vi "SetIndividualJoints.vi"(0 "Mode":T1=1 items=["Position"=1, "Velocity"=2, "Effort"=3], 1 "node":string, 2 "Joint States":T2(array[cluster]), 3 "error in":errorcluster) -> (6 "error out":errorcluster)   [LabVIEW 2012]
doc: "Set individual joints on Baxter"
uses:
  <userlib>/ROSforLV/ROS/Code/SubVIs/JointMode.ctl
  <userlib>/ROSforLV/ROS/Code/SubVIs/BaxterSide.ctl
  <userlib>/ROSforLV/ROS/Code/Console/Servers/ServerSubs/TopicDef.ctl
  <userlib>/ROSforLV/ROS/Code/SubVIs/_ROSDirection.ctl
  <userlib>/ROSforLV/ROS/MessageBuilding/std_msgs/subs/i32Scalar.vi
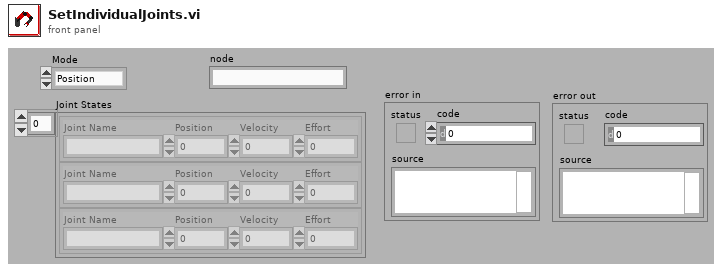
[diagram p1: front panel]
types:
  T1 = typedef "JointMode.ctl" = u8
  T2 = cluster{"Joint Name":string, "Position":dbl, "Velocity":dbl, "Effort":dbl}[]
  T3 = typedef "BaxterSide.ctl" = enum16{"left", "right"}
  T4 = typedef "TopicDef.ctl" = cluster{"Topic":string, "Type":string, "Action":T5, "Update (ms)":u16, "queue size":u16}
  T5 = typedef "_ROSDirection.ctl" = enum16{"Node", "Publisher", "Subscriber", "ServiceClient", "ServiceProvider"}
  T6 = typedef "_ROSControl.ctl" = cluster{"topic port":u16, "Node":string, "topic":string, "type":string, "node port":u16, "error ":errorcluster, "Direction":T5, "Update (ms)":u16, "FIFO size":u16}
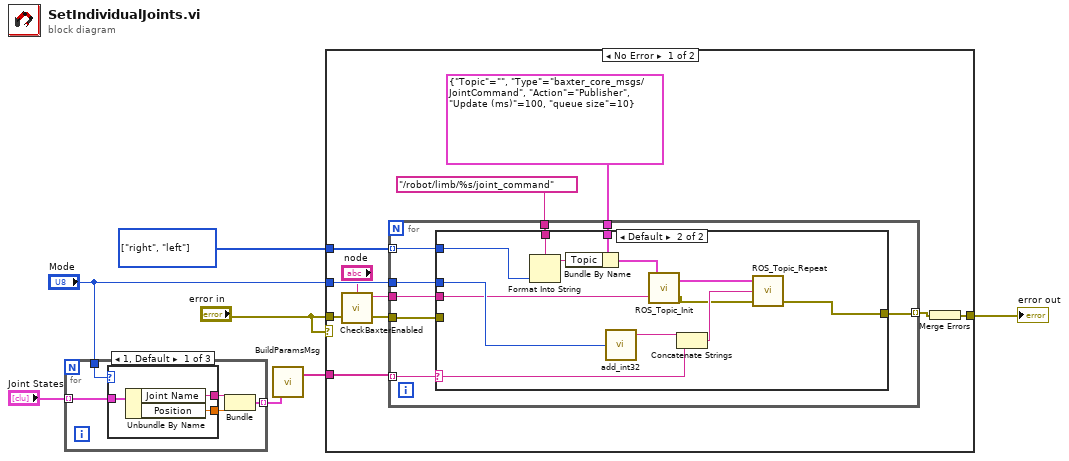
[diagram p0: block diagram]
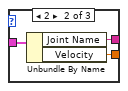
[diagram p4: hidden frame]
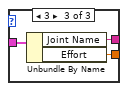
[diagram p5: hidden frame]
diagram:
  w7 = T3[] [enum."right", enum."left"] items=["left", "right"]
  n1 = for {
    tunnel: "Joint States" -> [w12] mode=indexing
    tunnel: "Mode" -> [w11]
    tunnel: [w8] -> w3 mode=indexing
    n2 = case shown="1, Default" w11 {
      tunnel: w12 -> [w15 w18 w21]
      tunnel: [w14 w17 w20] -> w10
      tunnel: [w13 w16 w19] -> w9
      frame 1, Default {
        n3 = Unbundle By Name(w15) -> ("Joint Name"=w14:string, "Position"=w13:dbl)
      }
      frame 2 {
        n4 = Unbundle By Name(w18) -> ("Joint Name"=w17:string, "Velocity"=w16:dbl)
      }
      frame 3 {
        n5 = Unbundle By Name(w21) -> ("Joint Name"=w20:string, "Effort"=w19:dbl)
      }
    }
    n6 = Bundle("Joint Name"=w10, "Effort"=w9) -> (w8:cluster{"Joint Name":string, "Effort":dbl})  [unwired: 1 in]
  }
  n7 = call <userlib>:"BuildParamsMsg.vi"("Parameters"=w3) -> ("Commands"=w2:string[])  [unwired: 1 in]
  n8 = case shown="No Error" "error in" {
    tunnel: w7 -> [w31 _]
    tunnel: [w30 w54] -> w6
    tunnel: "Mode" -> [w27 _]
    tunnel: w2 -> [w25 _]
    tunnel: "error in" -> [w24 w54]
    frame No Error {
      n9 = call <userlib>:"CheckBaxterEnabled.vi"("error in"=w24, "node"="node") -> ("error out"=w23:errorcluster)  [unwired: 2 in]
      n10 = for {
        tunnel: [w39] -> w29 mode=indexing
        tunnel: w23 -> [w38]
        tunnel: w31 -> [w37] mode=indexing
        tunnel: w27 -> [w36]
        tunnel: w25 -> [w35] mode=indexing
        tunnel: "/robot/limb/%s/joint_command" ("topic") -> [w34]
        tunnel: T4 {"Topic"="", "Type"="baxter_core_msgs/JointCommand", "Action"=enum."Publisher", "Update (ms)"=100, "queue size"=10} ("Definitions") -> [w33]
        tunnel: "node" -> [w32]
        n11 = case shown="Default" w35 {
          selector: w35 -> [_ w45]
          tunnel: [w40 w41] -> w39
          tunnel: w38 -> [w40 _]
          tunnel: w37 -> [_ w52]
          tunnel: w36 -> [_ w47]
          tunnel: w34 -> [_ w51]
          tunnel: w33 -> [_ w49]
          tunnel: w32 -> [_ w44]
          frame "" {
          }
          frame Default {
            n12 = Format Into String(format string=w51, w52) -> (resulting string=w50:string)  [unwired: 2 in, 1 out]
            n13 = Bundle By Name(cluster=w49, "Topic"=w50) -> (w48:T4)
            n14 = call-poly <userlib>:"add_int32.vi"("Numeric"=w47) -> ("msg out"=w46:string)  [unwired: 4 in]
            n15 = call <userlib>:"ROS_Topic_Init.vi"("node"=w44, "Definitions"=w48) -> ("error out"=w42:errorcluster, "ROS out"=w53:T6)
            n16 = Concatenate Strings(w46, w45) -> (w43:string)
            n17 = call <userlib>:"ROS_Topic_Repeat.vi"("error in (no error)"=w42, "Msg in"=w43, "ROS in"=w53) -> ("error out"=w41:errorcluster)  [unwired: 1 in, 1 out]
          }
        }
      }
      n18 = Merge Errors(w29) -> (w30:errorcluster)
    }
    frame Error {
    }
  }
  "error out" <- w6
